vi "LV_OPC_Test.vi"() -> ()   [LabVIEW 2018]
uses:
  OPC.DLL/LV_OPC.lvlib
panel:
  out "DBL":dbl=0.25
  out "SGL":sgl=0.1
  out "[Items]":string[](array[string])=["  0: '\\\\.\\Variables\\DBL'", "  1: '\\\\.\\Variables\\INT'", "  2: '\\\\.\\Variables\\SGL'"]
  out "Servers":string[](array[string])=["0: 'National Instruments.Variable Engine.1'", "1: 'National Instruments.NIOPCServers.V5'"]
  # "! Don't forget to deploy variables:"
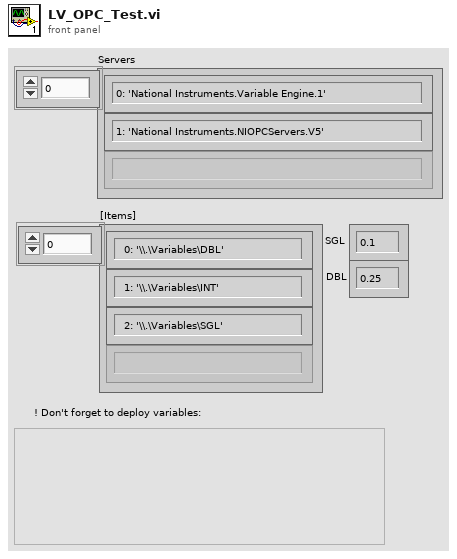
[diagram p1: front panel]
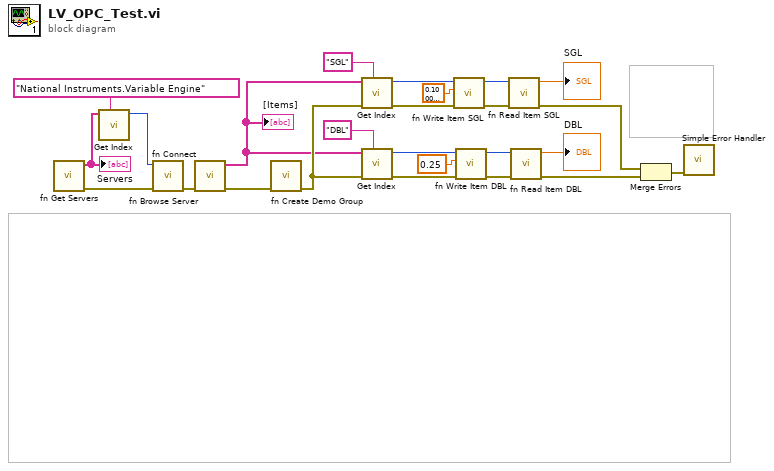
[diagram p0: block diagram]
diagram:
  n1 = call "fn Get Servers.vi"() -> ("error out"=w24:errorcluster, "[Servers]"=w22:string[])  [unwired: 10 in]
  "Servers" <- w22
  n2 = call "Get Index.vi"("item"="National Instruments.Variable Engine" ("regular expression"), "[Items]"=w22) -> ("index"=w25:i32)  [unwired: 8 in, 1 out]
  n3 = call "fn Connect.vi"("error in (no error)"=w24, "server_id"=w25) -> ("error out"=w23:errorcluster)  [unwired: 8 in, 1 out]
  n4 = call "fn Browse Server.vi"("error in (no error)"=w23) -> ("error out"=w21:errorcluster, "[Items]"=w19:string[])  [unwired: 9 in]
  "[Items]" <- w19
  n5 = call "fn Create Demo Group.vi"("error in (no error)"=w21) -> ("error out"=w20:errorcluster)  [unwired: 9 in, 1 out]
  n6 = call "Get Index.vi"("item"="SGL", "error in"=w20, "[Items]"=w19) -> ("error out"=w6:errorcluster, "index"=w14:i32)  [unwired: 7 in]
  n7 = call "Get Index.vi"("item"="DBL", "error in"=w20, "[Items]"=w19) -> ("error out"=w5:errorcluster, "index"=w15:i32)  [unwired: 7 in]
  n8 = call "fn Write Item SGL.vi"("error in (no error)"=w6, "val"=sgl 0.1, "idx"=w14) -> ("error out"=w4:errorcluster, "idx out (dup)"=w12:i32)  [unwired: 7 in]
  n9 = call "fn Write Item DBL.vi"("error in (no error)"=w5, "val"=0.25, "idx"=w15) -> ("error out"=w10:errorcluster, "idx out (dup)"=w8:i32)  [unwired: 7 in]
  n10 = call "fn Read Item SGL.vi"("error in (no error)"=w4, "idx"=w12) -> ("error out"=w3:errorcluster, "function return"=→"SGL":sgl)  [unwired: 8 in]
  n11 = call "fn Read Item DBL.vi"("error in (no error)"=w10, "idx"=w8) -> ("error out"=w2:errorcluster, "function return"=→"DBL":dbl)  [unwired: 8 in]
  n12 = Merge Errors(w3, w2) -> (w1:errorcluster)
  n13 = call <vilib>:"Simple Error Handler.vi"("error in (no error)"=w1) -> ()  [unwired: 4 in, 5 out]
